vi "FGV_GitData.vi"(5 "Enum":enum16{"Set", "Get"}(ring), 9 "Git Commit Array Input":T1[](array[typedef])) -> (3 "Git Commit Array Output":T1[](array[typedef]))   [LabVIEW 2018, in "feGEM DataPacker.lvlib"]
uses:
  feGEM DataPacker.lvlib
  GitTools/GitCommitData.ctl
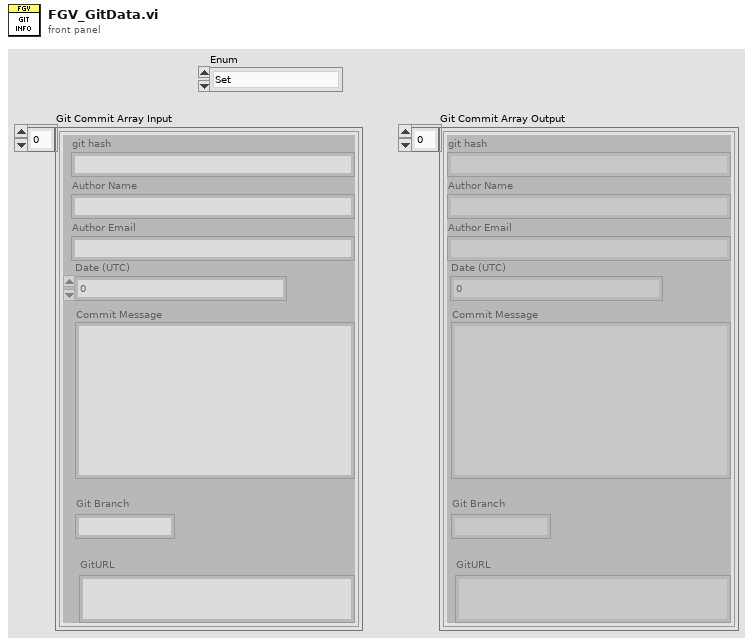
[diagram p1: front panel]
types:
  T1 = typedef "feGEM DataPacker.lvlib/GitCommitData.ctl" = cluster{"git hash":string, "Author Name":string, "Author Email":string, "Date (UTC)":i32, "Commit Message":string, "GitURL":string, "Git Branch":string}
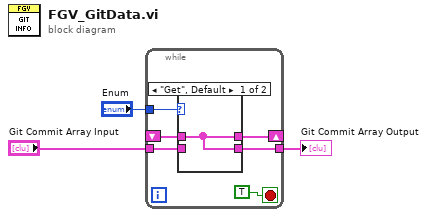
[diagram p0: block diagram]
diagram:
  n1 = while {
    shift-right: [w8] -> _
    shift-left: _ -> [w9]
    tunnel: "Git Commit Array Input" -> [w6]
    tunnel: [w7] -> w2
    tunnel: "Enum" -> [w5]
    stop <- TRUE stop-if-true
    n2 = case shown="\"Get\", Default" w5 {
      tunnel: [w10 w11] -> w7
      tunnel: [w10 w11] -> w8
      tunnel: w9 -> [w10 _]
      tunnel: w6 -> [_ w11]
      frame "Get", Default {
      }
      frame "Set" {
      }
    }
  }
  "Git Commit Array Output" <- w2
